vi "comparison.vi"() -> ()   [LabVIEW 2016]
panel:
  in  "stop":bool
  out "Equal":bool
  in  "Number2":dbl
  in  "Number1":dbl
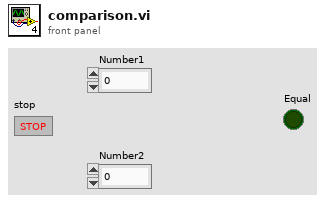
[diagram p1: front panel]
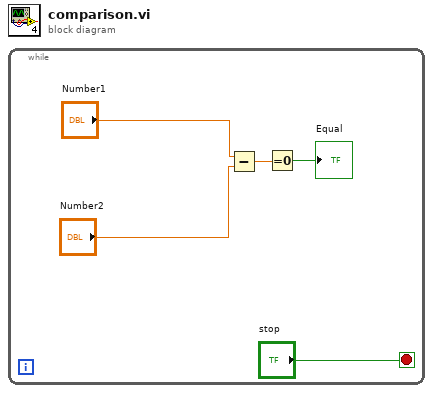
[diagram p0: block diagram]
diagram:
  n1 = while {
    stop <- "stop" stop-if-true
    n2 = Subtract(x="Number1", y="Number2") -> (x-y=w3:dbl)
    n3 = Equal To 0?(x=w3) -> (x = 0?=→"Equal":bool)
  }
